vi "例4.20-1求方程的根.vi"() -> ()   [LabVIEW 2012]
panel:
  out "x2":dbl
  out "x1":dbl
  in  "c":dbl
  in  "b":dbl
  in  "a":dbl
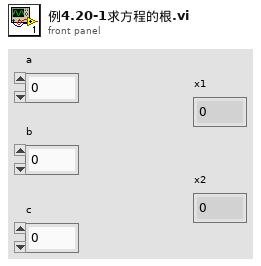
[diagram p1: front panel]
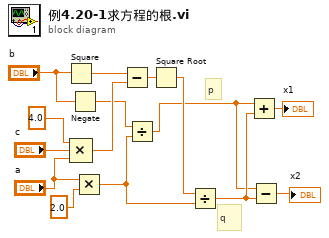
[diagram p0: block diagram]
diagram:
  # "p"
  # "q"
  n1 = Square(x="b") -> (x^2=w14:dbl)
  n2 = Negate(x="b") -> (-x=w10:dbl)
  n3 = Compound Arithmetic op=MULTIPLY(4.0 ("值"), "c", "a") -> (w13:dbl)
  n4 = Multiply(x="a", y=2.0) -> (x*y=w4:dbl)
  n5 = Subtract(x=w14, y=w13) -> (x-y=w9:dbl)
  n6 = Divide(x=w10, y=w4) -> (x/y=w1:dbl)
  n7 = Square Root(x=w9) -> (sqrt(x)=w8:dbl)
  n8 = Divide(x=w8, y=w4) -> (x/y=w6:dbl)
  n9 = Add(x=w1, y=w6) -> (x+y=→"x1":dbl)
  n10 = Subtract(x=w1, y=w6) -> (x-y=→"x2":dbl)
